vi "SPV.vi"(0 "System no.":i32=1 min=1 max=4 step=1, 2 "ParameterSet":T2, 5 "error in":errorcluster) -> (19 "error out":errorcluster)   [LabVIEW 2026]
doc: "Sets the value of a configuration parameter in a memory of the controller."
uses:
  MemoryType.ctl
  Parameter Set.ctl
panel:
  in  "Memory Type":T1
  # "Set a parameter value for defined Memory, ContainerUnit, FunctionUnit and ParameterID. In order to set a value the parameter set must be fully specified."
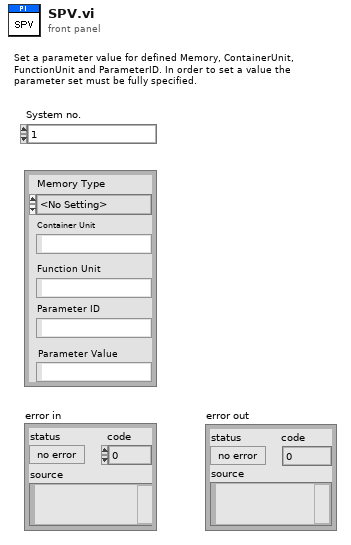
[diagram p1: front panel]
types:
  T1 = typedef "MemoryType.ctl" = enum16{"<No Setting>", "RAM", "FLASH", "TMP"}
  T2 = typedef "Parameter Set.ctl" = cluster{"Memory Type":T1, "Container Unit":string, "Function Unit":string, "Parameter ID":string, "Parameter Value":string}
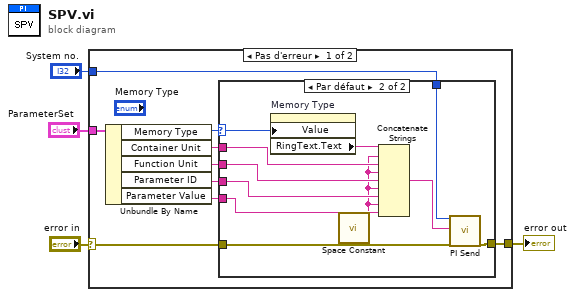
[diagram p0: block diagram]
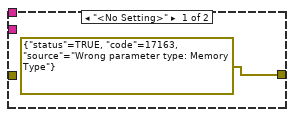
[diagram p2: hidden frame]
diagram:
  n1 = case shown="Pas d'erreur" "error in" {
    selector: "error in" -> [w13 w26]
    tunnel: "System no." -> [w12 _]
    tunnel: [w11 w26] -> w3
    tunnel: "ParameterSet" -> [w10 _]
    frame No Error {
      n2 = Unbundle By Name(w10) -> ("Memory Type"=w9:T1, "Container Unit"=w8:string, "Function Unit"=w7:string, "Parameter ID"=w6:string, "Parameter Value"=w5:string)
      n3 = case shown="Par défaut" w9 {
        selector: w9 -> [_ w25]
        tunnel: w13 -> [_ w16]
        tunnel: w12 -> [_ w18]
        tunnel: [errorcluster {"status"=TRUE, "code"=17163, "source"="Wrong parameter type: Memory Type"} ("error out") w15] -> w11
        tunnel: w8 -> [_ w23]
        tunnel: w7 -> [_ w22]
        tunnel: w6 -> [_ w21]
        tunnel: w5 -> [_ w20]
        frame "<No Setting>" {
        }
        frame Default {
          n4 = property on="Memory Type" class="Énum (strict)"("Value"=w25) -> ("RingText.Text"=w24:string)  [unwired: 2 in, 2 out]
          n5 = call <vilib>:"Space Constant.vi"() -> ("String"=w19:string)
          n6 = Concatenate Strings(w24, w19, w23, w19, w22, w19, w21, w19, w20) -> (w17:string)
          n7 = call "PI Send.vi"("System no."=w18, "String to send"=w17, "error in"=w16) -> ("error out"=w15:errorcluster)  [unwired: 15 in, 1 out]
        }
      }
    }
    frame Error {
    }
  }
  "error out" <- w3
